vi "_011.vi"() -> ()   [LabVIEW 2024]
panel:
  out "Numeric 3":dbl
  in  "stop":bool
  in  "Numeric 2":dbl
  out "Array":dbl[](array[numeric])
  in  "y":dbl
  in  "Numeric":dbl
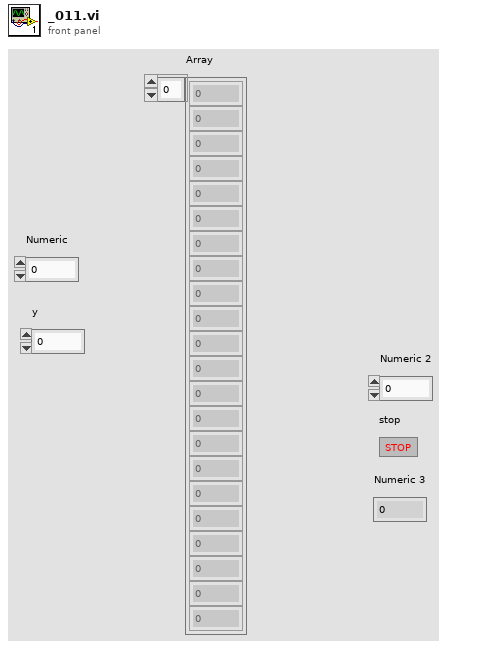
[diagram p1: front panel]
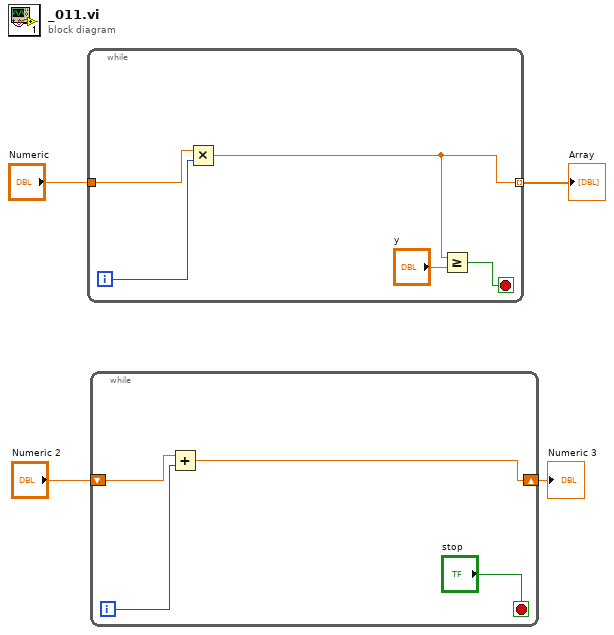
[diagram p0: block diagram]
diagram:
  n1 = while {
    tunnel: "Numeric" -> [w9]
    tunnel: [w5] -> w3 mode=indexing
    i -> [w8]
    stop <- w7 stop-if-true
    n2 = Multiply(x=w9, y=w8) -> (x*y=w5:dbl)
    n3 = Greater Or Equal?(x=w5, y="y") -> (x >= y?=w7:bool)
  }
  "Array" <- w3
  n4 = while {
    shift-right: [w12] -> w1
    shift-left: "Numeric 2" -> [w13]
    i -> [w11]
    stop <- "stop" stop-if-true
    n5 = Add(x=w13, y=w11) -> (x+y=w12:dbl)
  }
  "Numeric 3" <- w1
